vi "Swaps the source step with destination step for AUTO.vi"(8 "error in":errorcluster, 9 "Destination Step":u8=1 min=1 max=16, 10 "Source Step":u8=1 min=1 max=16, 11 "VISA resource name":refnum<visa-resource-name>) -> (0 "error out":errorcluster, 3 "VISA resource name out":refnum<visa-resource-name>)   [LabVIEW 2011, in "GPT-9000.lvlib"]
uses:
  <instrlib>/GPT-9000/GPT-9000.lvlib
panel:
  # "SWAP"
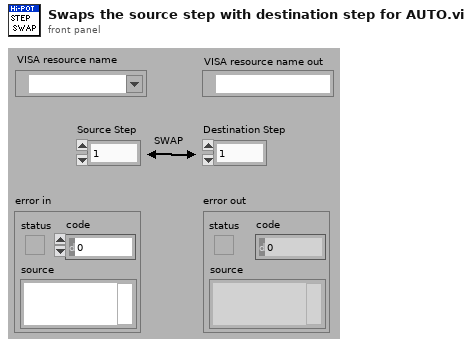
[diagram p1: front panel]
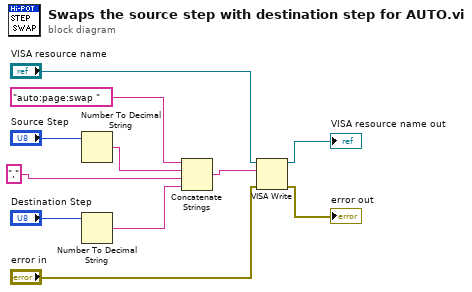
[diagram p0: block diagram]
diagram:
  n1 = Number To Decimal String(number="Source Step") -> (decimal integer string=w8:string)  [unwired: 1 in]
  n2 = Number To Decimal String(number="Destination Step") -> (decimal integer string=w6:string)  [unwired: 1 in]
  n3 = Concatenate Strings("auto:page:swap ", w8, ",", w6) -> (w3:string)
  n4 = VISA Write(VISA resource name="VISA resource name", write buffer=w3, error in (no error)="error in") -> (VISA resource name out=→"VISA resource name out":refnum<visa-resource-name>, error out=→"error out":errorcluster)  [unwired: 1 out]
